vi "Agilent DMM Read Range.vi"(7 "Measurement Type":T2, 8 "error in (no error)":errorcluster, 11 "VISA Resource Name":refnum<visa-resource-name>) -> (0 "error out":errorcluster, 2 "Range":T1, 3 "dup VISA Resource Name":refnum<visa-resource-name>)   [LabVIEW 2011]
doc: "This VI for the HP 8753 is used to read the sweep type.\n\n0 LINEAR FREQ\n1 LOG FREQ\n2 LIST FREQ\n3 CW TIME\n4 POWER SWEEP"
uses:
  TypeDefs/Agilent DMM Measurement Type.ctl
  TypeDefs/Agilent DMM Range.ctl
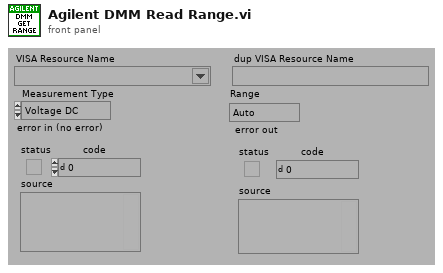
[diagram p1: front panel]
types:
  T1 = typedef "Agilent DMM Range.ctl" = enum16{"Auto", "Min", "Max", "0.01", "0.1", "1", "3", "10", "100", "1,000", "10,000", "100,000", "1,000,000", "10,000,000", "100,000,000"}
  T2 = typedef "Agilent DMM Measurement Type.ctl" = enum16{"Voltage DC", "Voltage DC Ratio", "Voltage AC", "Current DC", "Current AC", "Resistance", "Fresistance", "Frequency", "Period", "Continuity", "Diode"}
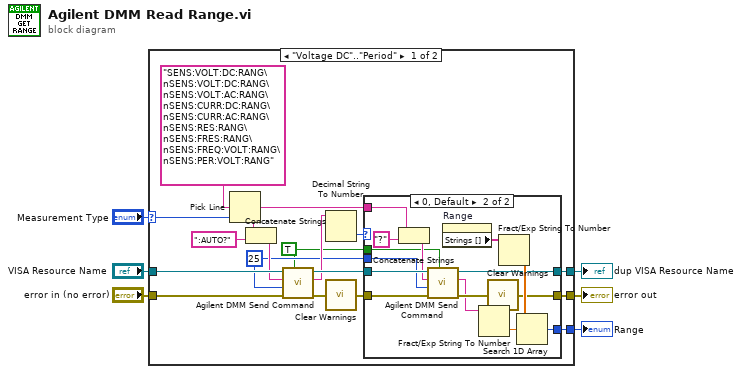
[diagram p0: block diagram]
diagram:
  n1 = case shown="\"Voltage DC\"..\"Period\"" "Measurement Type" {
    selector: "Measurement Type" -> [w22 _]
    tunnel: "error in (no error)" -> [w16 w42]
    tunnel: [w21 w42] -> w5
    tunnel: "VISA Resource Name" -> [w17 w41]
    tunnel: [w20 w41] -> w3
    tunnel: [w14 _] -> w1
    frame "Voltage DC".."Period" {
      w7 = TRUE ("Read? (F)")
      w8 = u32 25
      n2 = Pick Line(multi-line string="SENS:VOLT:DC:RANG\nSENS:VOLT:DC:RANG\nSENS:VOLT:AC:RANG\nSENS:CURR:DC:RANG\nSENS:CURR:AC:RANG\nSENS:RES:RANG\nSENS:FRES:RANG\nSENS:FREQ:VOLT:RANG\nSENS:PER:VOLT:RANG" ("write buffer"), line index=w22) -> (output string=w19:string)  [unwired: 1 out]
      n3 = Concatenate Strings(w19, ":AUTO?" ("string")) -> (w15:string)
      n4 = call "Agilent DMM Send Command.vi"("Read? (F)"=w7, "error in (no error)"=w16, "Byte Count"=w8, "Command"=w15, "VISA Resource Name"=w17) -> ("error out"=w9:errorcluster, "Data Read"=w10:string, "dup VISA Resource Name"=w11:refnum<visa-resource-name>)  [unwired: 4 out]
      n5 = Decimal String To Number(string=w10) -> (number=w13:i32)  [unwired: 3 out]
      n6 = call "Clear Warnings.vi"("error in (no error)"=w9) -> ("error out"=w12:errorcluster)
      n7 = case shown="0, Default" w13 {
        tunnel: w12 -> [w24 w40]
        tunnel: w11 -> [w25 w39]
        tunnel: w19 -> [_ w38]
        tunnel: [w24 w31] -> w21
        tunnel: [w25 w28] -> w20
        tunnel: w8 -> [_ w29]
        tunnel: [_ w32] -> w14
        tunnel: w7 -> [_ w26]
        frame 1 {
        }
        frame 0, Default {
          n8 = Concatenate Strings(w38, "?" ("string")) -> (w37:string)
          n9 = call "Agilent DMM Send Command.vi"("Read? (F)"=w26, "error in (no error)"=w40, "Byte Count"=w29, "Command"=w37, "VISA Resource Name"=w39) -> ("error out"=w30:errorcluster, "Data Read"=w27:string, "dup VISA Resource Name"=w28:refnum<visa-resource-name>)  [unwired: 4 out]
          n10 = property on="Range" class="Enum (strict)"() -> ("Strings []"=w35:string[])  [unwired: 2 in, 2 out]
          n11 = Fract/Exp String To Number(string=w27) -> (number=w33:dbl)  [unwired: 4 out]
          n12 = call "Clear Warnings.vi"("error in (no error)"=w30) -> ("error out"=w31:errorcluster)
          n13 = Fract/Exp String To Number(string=w35) -> (number=w34:dbl[])  [unwired: 4 out]
          n14 = Search 1D Array(1D array=w34, element=w33) -> (index of element=w32:i32)  [unwired: 1 out]
        }
      }
    }
    frame Default {
      # "The Range can not be read for:\n\nContinuity, or Diode."
    }
  }
  "dup VISA Resource Name" <- w3
  "error out" <- w5
  "Range" <- w1
